vi "Set Control Value and Signal Value.vi"(8 "错误输入（无错误）":errorcluster, 9 "Mode":enum16{"Set Value", "Set Signal Value"}(ring), 10 "Value":variant, 11 "Ctl Ref In":refnum<vi>) -> (0 "错误输出":errorcluster, 3 "Ctl Ref Out":refnum<vi>)   [LabVIEW 2012, in "CtrlRef.lvlib"]
uses:
  CtrlRef.lvlib
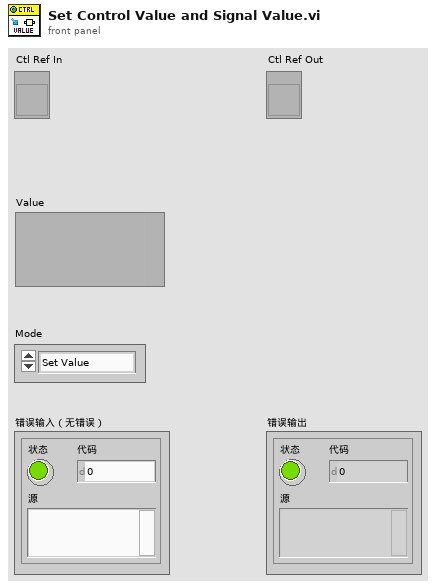
[diagram p1: front panel]
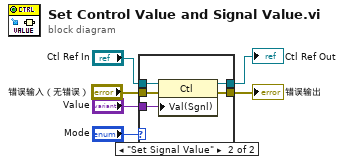
[diagram p0: block diagram]
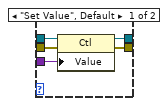
[diagram p2: hidden frame]
diagram:
  n1 = case shown="\"Set Signal Value\"" "Mode" {
    tunnel: "错误输入（无错误）" -> [w11 w15]
    tunnel: "Ctl Ref In" -> [w10 w16]
    tunnel: [w9 w13] -> w3
    tunnel: [w8 w12] -> w1
    tunnel: "Value" -> [w7 w14]
    frame "Set Value", Default {
      n2 = property class="Ctl"(reference=w10, error in=w11, "Value"=w7) -> (reference out=w9:refnum<vi>, error out=w8:errorcluster)
    }
    frame "Set Signal Value" {
      n3 = property class="Ctl"(reference=w16, error in=w15, "Val(Sgnl)"=w14) -> (reference out=w13:refnum<vi>, error out=w12:errorcluster)
    }
  }
  "错误输出" <- w1
  "Ctl Ref Out" <- w3
